vi "Miniquads.add services.vi"(0 "i ref in":refnum<vi>, 3 "ms timeout (10000)":i32=10000, 5 "error in (no error)":errorcluster) -> (14 "i ref out":refnum<vi>, 17 "timed out":bool, 19 "error out":errorcluster)   [LabVIEW 2014, in "Miniquads.lvlib"]
doc: "Declares the required DIM services."
uses:
  Miniquads.lvlib
  CSlibraries-extern/DimLVEvent/LVDimInterface/LVDimInterface.lvlib
  CSCore/CSSystem/CSSystemLib/CSSystemLib.lvlib
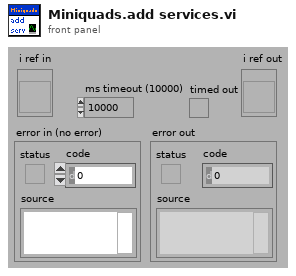
[diagram p1: front panel]
types:
  T1 = typedef "Miniquads.lvlib/Miniquads.i attribute.ctl" = cluster{"ObjectsInitialized":bool, "ObjectsLoaded":string[], "nomValues":T2, "actValues":T2}
  T2 = typedef "Miniquads.lvlib/Miniquads.voltages.ctl" = cluster{"FocusVoltage":dbl, "HorizontalVoltage":dbl, "VerticalVoltage":dbl, "serviceIDs":cluster{"FocusVoltageID":i32, "HorizontalVoltageID":i32, "VerticalVoltageID":i32}}
  T3 = cluster{"my_serviceID":i32, "my_serviceID":i32, "my_serviceID":i32}
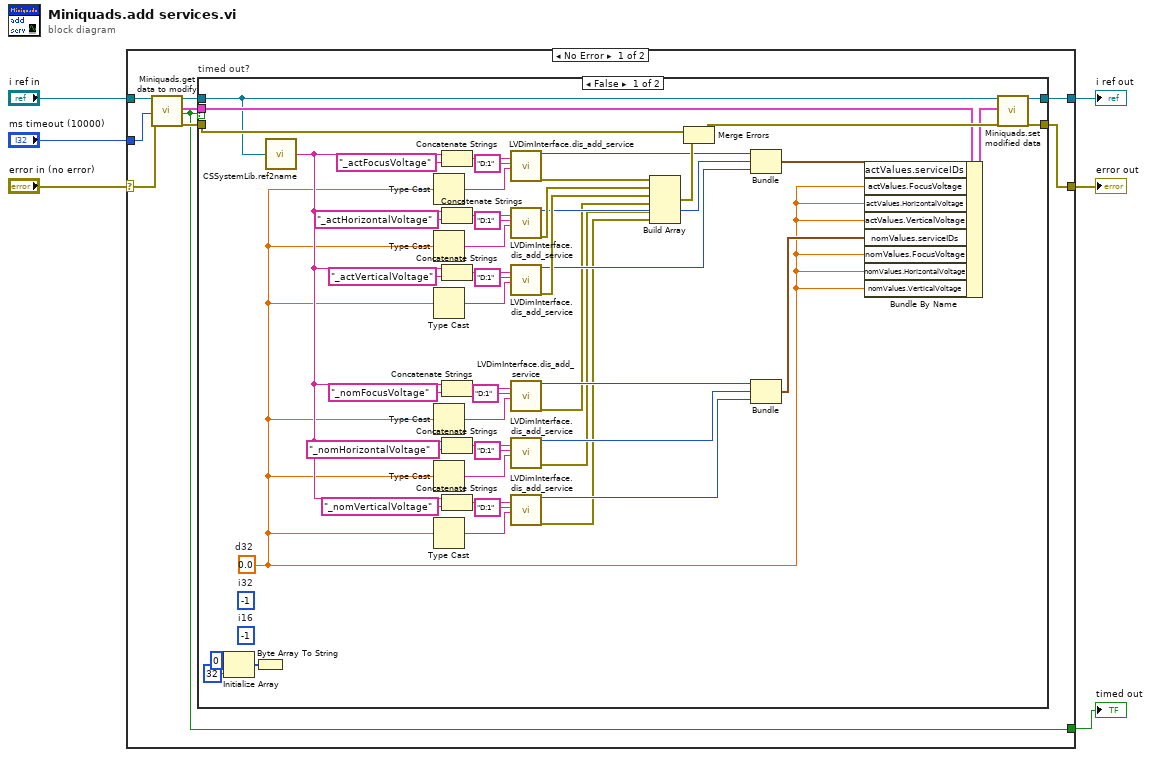
[diagram p0: block diagram]
diagram:
  n1 = case shown="No Error" "error in (no error)" {
    selector: "error in (no error)" -> [w13 w70]
    tunnel: [w9 w70] -> w5
    tunnel: "i ref in" -> [w15 w69]
    tunnel: [w11 w69] -> w3
    tunnel: "ms timeout (10000)" -> [w14 _]
    tunnel: [w8 _] -> w1
    frame No Error {
      n2 = call "Miniquads.get data to modify.vi"("i ref in"=w15, "ms timeout (10000)"=w14, "error in (no error)"=w13) -> ("i ref out"=w12:refnum<vi>, "i attribute"=w7:T1, "timed out"=w8:bool, "error out"=w10:errorcluster)  [unwired: 13 in]
      n3 = case "timed out?" shown="False" w8 {
        tunnel: w12 -> [w26 w68]
        tunnel: [w66 w68] -> w11
        tunnel: w10 -> [w37 w67]
        tunnel: [w65 w67] -> w9
        tunnel: w7 -> [w34 _]
        frame False {
          w16 = 0.0  # d32
          (unwired) i16 -1  # i16
          (unwired) -1  # i32
          n4 = Initialize Array(u8 0, 32 ("dimension size")) -> (w23:u8[])
          n5 = Byte Array To String(unsigned byte array=w23) -> ()  [unwired: 1 out]
          n6 = call "CSSystemLib.ref2name.vi"("obj refnum"=w26) -> ("name"=w20:string)
          n7 = Type Cast(x=w16) -> (*(type *) &x=w61:string)  [unwired: 1 in]
          n8 = Type Cast(x=w16) -> (*(type *) &x=w60:string)  [unwired: 1 in]
          n9 = Type Cast(x=w16) -> (*(type *) &x=w53:string)  [unwired: 1 in]
          n10 = Type Cast(x=w16) -> (*(type *) &x=w49:string)  [unwired: 1 in]
          n11 = Type Cast(x=w16) -> (*(type *) &x=w48:string)  [unwired: 1 in]
          n12 = Type Cast(x=w16) -> (*(type *) &x=w41:string)  [unwired: 1 in]
          n13 = Concatenate Strings(w20, "_actFocusVoltage" ("string")) -> (w64:string)
          n14 = Concatenate Strings(w20, "_actHorizontalVoltage" ("string")) -> (w57:string)
          n15 = Concatenate Strings(w20, "_actVerticalVoltage" ("string")) -> (w56:string)
          n16 = Concatenate Strings(w20, "_nomFocusVoltage" ("string")) -> (w52:string)
          n17 = Concatenate Strings(w20, "_nomHorizontalVoltage" ("string")) -> (w45:string)
          n18 = Concatenate Strings(w20, "_nomVerticalVoltage" ("string")) -> (w44:string)
          n19 = call "LVDimInterface.dis_add_service.vi"("serviceName"=w64, "typeDescriptor"="D:1", "data"=w61) -> ("my_serviceID"=w33:i32, "error out"=w40:errorcluster)  [unwired: 15 in]
          n20 = call "LVDimInterface.dis_add_service.vi"("serviceName"=w57, "typeDescriptor"="D:1", "data"=w60) -> ("my_serviceID"=w32:i32, "error out"=w39:errorcluster)  [unwired: 15 in]
          n21 = call "LVDimInterface.dis_add_service.vi"("serviceName"=w56, "typeDescriptor"="D:1", "data"=w53) -> ("my_serviceID"=w31:i32, "error out"=w38:errorcluster)  [unwired: 15 in]
          n22 = call "LVDimInterface.dis_add_service.vi"("serviceName"=w52, "typeDescriptor"="D:1", "data"=w49) -> ("my_serviceID"=w30:i32, "error out"=w19:errorcluster)  [unwired: 15 in]
          n23 = call "LVDimInterface.dis_add_service.vi"("serviceName"=w45, "typeDescriptor"="D:1", "data"=w48) -> ("my_serviceID"=w29:i32, "error out"=w18:errorcluster)  [unwired: 15 in]
          n24 = call "LVDimInterface.dis_add_service.vi"("serviceName"=w44, "typeDescriptor"="D:1", "data"=w41) -> ("my_serviceID"=w28:i32, "error out"=w17:errorcluster)  [unwired: 15 in]
          n25 = Build Array(w40, w39, w38, w19, w18, w17) -> (w36:errorcluster[])
          n26 = Merge Errors(w37, w36) -> (w35:errorcluster)
          n27 = Bundle("my_serviceID"=w33, "my_serviceID"=w32, "my_serviceID"=w31) -> (w24:T3)  [unwired: 1 in]
          n28 = Bundle("my_serviceID"=w30, "my_serviceID"=w29, "my_serviceID"=w28) -> (w25:T3)  [unwired: 1 in]
          n29 = Bundle By Name(cluster=w34, "actValues.serviceIDs"=w24, "actValues.FocusVoltage"=w16, "actValues.HorizontalVoltage"=w16, "actValues.VerticalVoltage"=w16, "nomValues.serviceIDs"=w25, "nomValues.FocusVoltage"=w16, "nomValues.HorizontalVoltage"=w16, "nomValues.VerticalVoltage"=w16) -> (w27:T1)
          n30 = call "Miniquads.set modified data.vi"("i ref in"=w26, "i attribute"=w27, "error in (no error)"=w35) -> ("i ref out"=w66:refnum<vi>, "error out"=w65:errorcluster)  [unwired: 15 in]
        }
        frame True {
        }
      }
    }
    frame Error {
    }
  }
  "error out" <- w5
  "i ref out" <- w3
  "timed out" <- w1
